vi "mod.Test2.vi"(8 "error in":errorcluster, 10 "Data":variant, 11 "Command":string) -> (0 "error out":errorcluster, 3 "Return Data":variant)   [LabVIEW 2014]
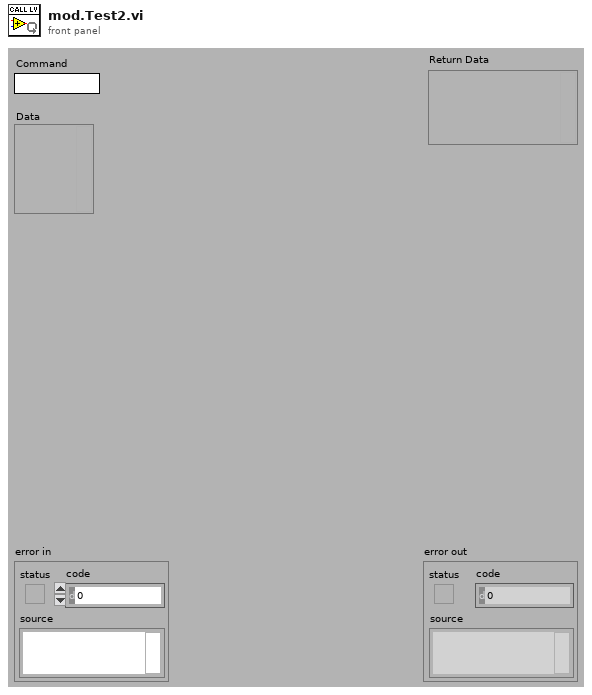
[diagram p1: front panel]
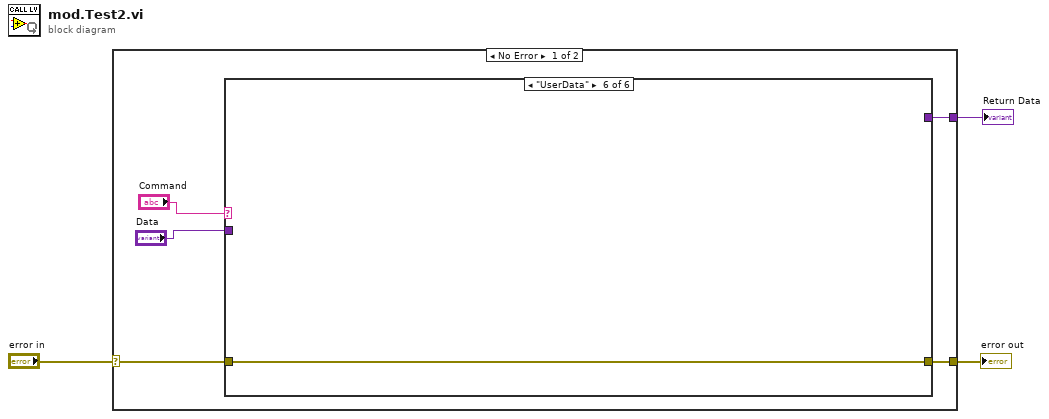
[diagram p0: block diagram]
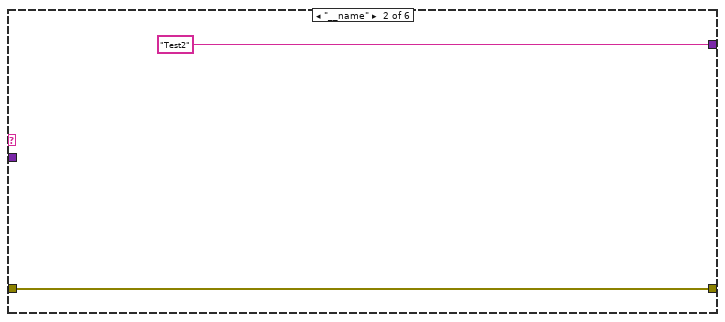
[diagram p3: hidden frame]
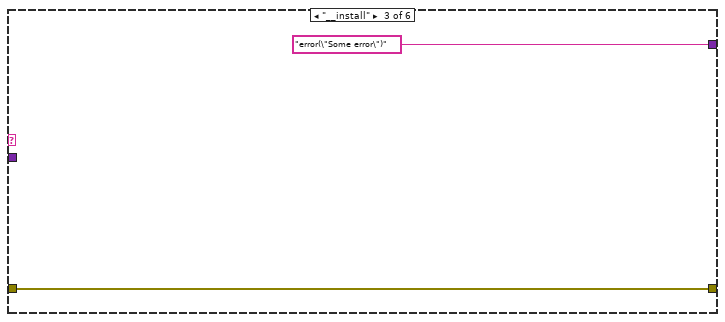
[diagram p4: hidden frame]
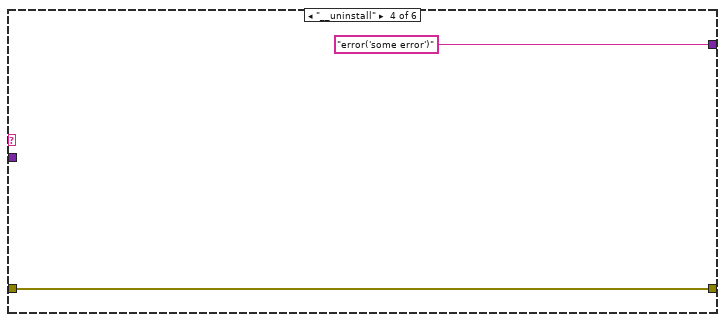
[diagram p5: hidden frame]
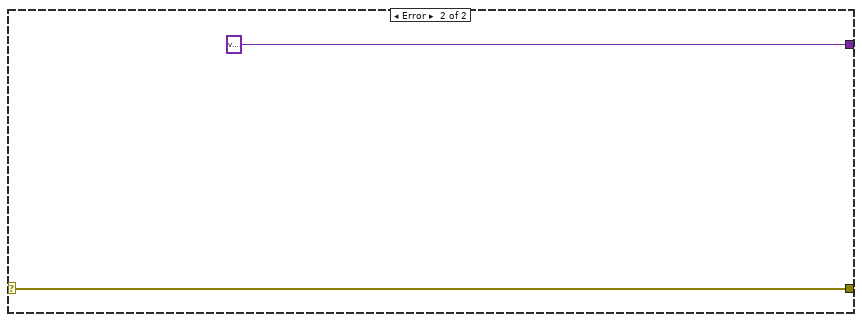
[diagram p7: hidden frame]
diagram:
  n1 = case shown="No Error" "error in" {
    selector: "error in" -> [w8 w21]
    tunnel: [w6 w21] -> w2
    tunnel: [w7 variant ("User Data")] -> w1
    frame No Error {
      n2 = case shown="\"UserData\"" "Command" {
        tunnel: w8 -> [w10 w11 w13 w15 w18 w19]
        tunnel: "Data" -> [w9 _ _ _ w17 _]
        tunnel: [w9 "Test2" "error(\"Some error\")" "error('some error')" w17 _] -> w7
        tunnel: [w10 w11 w13 w15 w18 w19] -> w6
        frame Default {
        }
        frame "__name" {
        }
        frame "__install" {
        }
        frame "__uninstall" {
        }
        frame "PassThrough" {
        }
        frame "UserData" {
        }
      }
    }
    frame Error {
    }
  }
  "Return Data" <- w1
  "error out" <- w2
